vi "XY graph.vi"() -> ()   [LabVIEW 2014]
panel:
  out "Y":dbl
  out "X":dbl
  in  "stop":bool
  out "XY Graph":cluster{"X":dbl, "Y":dbl}[](graph)
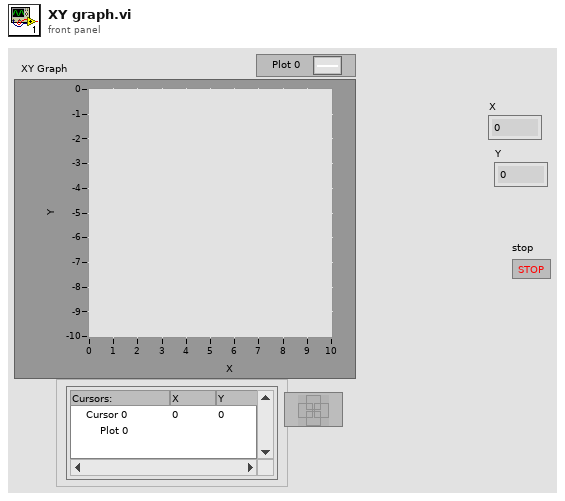
[diagram p1: front panel]
types:
  T1 = typedef "LVPointDoubleTypeDef.ctl" = cluster{"Cursor X":dbl, "Cursor Y":dbl}
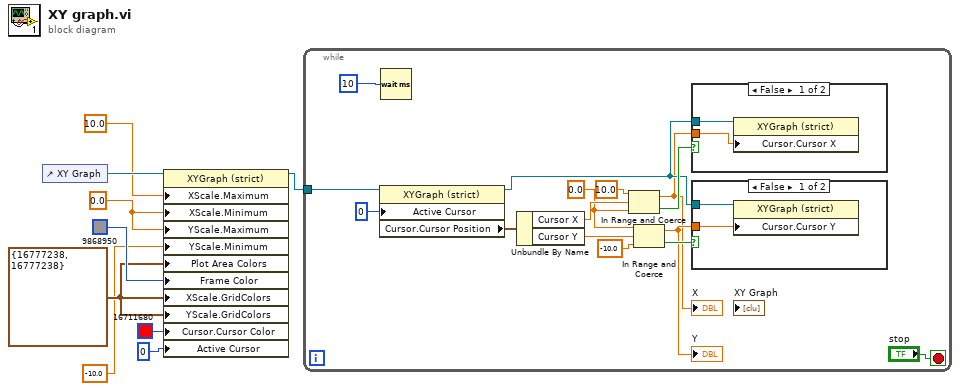
[diagram p0: block diagram]
diagram:
  w6 = cluster{u32, u32} {16777238, 16777238}
  w3 = 0.0
  n1 = control-ref of="XY Graph"() -> (w9:refnum<vi>)
  n2 = property class="XYGraph (strict)"(reference=w9, "XScale.Maximum"=10.0, "XScale.Minimum"=w3, "YScale.Maximum"=w3, "YScale.Minimum"=-10.0, "Plot Area Colors"=w6, "Frame Color"=u32 9868950, "XScale.GridColors"=w6, "YScale.GridColors"=w6, "Cursor.Cursor Color"=u32 16711680, "Active Cursor"=u32 0) -> (reference out=w8:refnum<vi>)  [unwired: 1 in, 1 out]
  n3 = while {
    tunnel: w8 -> [w23]
    stop <- "stop" stop-if-true
    w18 = 0.0
    n4 = property class="XYGraph (strict)"(reference=w23, "Active Cursor"=0) -> (reference out=w12:refnum<vi>, "Cursor.Cursor Position"=w17:T1)  [unwired: 1 in, 1 out]
    n5 = Wait (ms)(milliseconds to wait=10) -> ()  [unwired: 1 out]
    n6 = Unbundle By Name(w17) -> ("Cursor X"=w22:dbl, "Cursor Y"=w20:dbl)
    n7 = In Range and Coerce(upper limit=10.0, x=w22, lower limit=w18) -> (coerced(x)=w10:dbl, In Range?=w14:bool)
    "X" <- w10
    n8 = In Range and Coerce(upper limit=w18, x=w20, lower limit=-10.0) -> (coerced(x)=w11:dbl, In Range?=w13:bool)
    "Y" <- w11
    n9 = case shown="False" w14 {
      tunnel: w12 -> [w28 _]
      tunnel: w10 -> [w27 _]
      frame False {
        n10 = property class="XYGraph (strict)"(reference=w28, "Cursor.Cursor X"=w27) -> ()  [unwired: 1 in, 2 out]
      }
      frame True {
      }
    }
    n11 = case shown="False" w13 {
      tunnel: w12 -> [w26 _]
      tunnel: w11 -> [w25 _]
      frame False {
        n12 = property class="XYGraph (strict)"(reference=w26, "Cursor.Cursor Y"=w25) -> ()  [unwired: 1 in, 2 out]
      }
      frame True {
      }
    }
  }
